vi "rot3d to Memory Cell.vi"(10 "Orient3d in":refnum<class "Orient3d Class.lvclass">) -> (2 "Memory Cell":T1={"type"=enum."vector", "x"=0.0, "y"=0.0, "z"=0.0, "w"=0.0})   [LabVIEW 2017]
uses:
  Type Definitions/Memory Cell.ctl
  Type Definitions/Memory Cell Type Enum.ctl
  Shared Components/Orient3d Class/Orient3d Class.lvclass
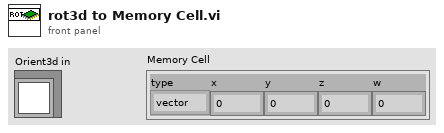
[diagram p1: front panel]
types:
  T1 = typedef "Memory Cell.ctl" = cluster{"type":T2, "x":dbl, "y":dbl, "z":dbl, "w":dbl}
  T2 = typedef "Memory Cell Type Enum.ctl" = enum16{"integer", "float", "vector", "rotation"}
  T3 = typedef "Quaternion.ctl" = cluster{"x":dbl, "y":dbl, "z":dbl, "w":dbl}
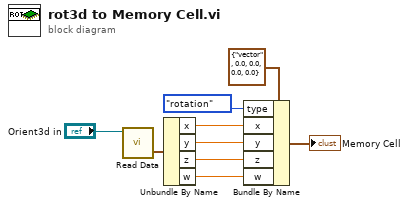
[diagram p0: block diagram]
diagram:
  n1 = call "Read Data.vi"("Orient3d in"="Orient3d in") -> ("Quaternion"=w5:T3)  [unwired: 8 in, 2 out]
  n2 = Unbundle By Name(w5) -> ("x"=w4:dbl, "y"=w3:dbl, "z"=w2:dbl, "w"=w1:dbl)
  n3 = Bundle By Name(cluster=T1 {"type"=enum."vector", "x"=0.0, "y"=0.0, "z"=0.0, "w"=0.0} ("Memory Cell 2"), "type"=Memory_Cell_Type_Enum."rotation", "x"=w4, "y"=w3, "z"=w2, "w"=w1) -> (→"Memory Cell":T1)
